vi "div10.vi"(1 "x":dbl) -> (0 "y":dbl)   [LabVIEW 2022 SP3]
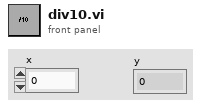
[diagram p1: front panel]
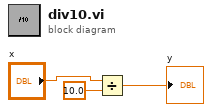
[diagram p0: block diagram]
diagram:
  n1 = Divide(x="x", y=10.0) -> (x/y=→"y":dbl)
